vi "Read Buffered Data.vi"(8 "error in (no error)":errorcluster, 11 "Standard Measurement in":refnum<class "Standard Measurement.lvclass">) -> (0 "error out":errorcluster, 3 "Standard Measurement out":refnum<class "Standard Measurement.lvclass">)   [LabVIEW 2026, in "Standard Measurement Plugin.lvlib" / "Standard Measurement.lvclass"]
doc: "Read one snapshot from each configured Standard Measurement hardware buffer and store latest waveforms. Three hardware roles maximum; each preview waits at most 1 ms, zero retries. Incoming errors bypass reads through the framework accessors; timeout or type conversion errors propagate. No hardware initialization or actor launch."
uses:
  Standard Measurement.lvclass
  framework/Measurement Actor/Measurement.lvclass
  framework/Hardware/Hardware.lvclass
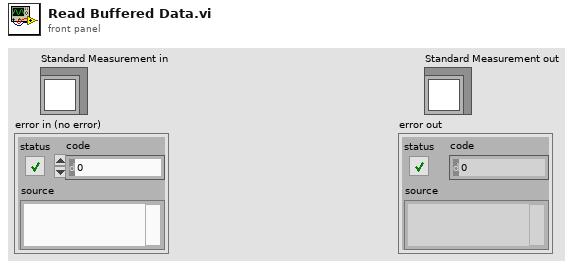
[diagram p1: front panel]
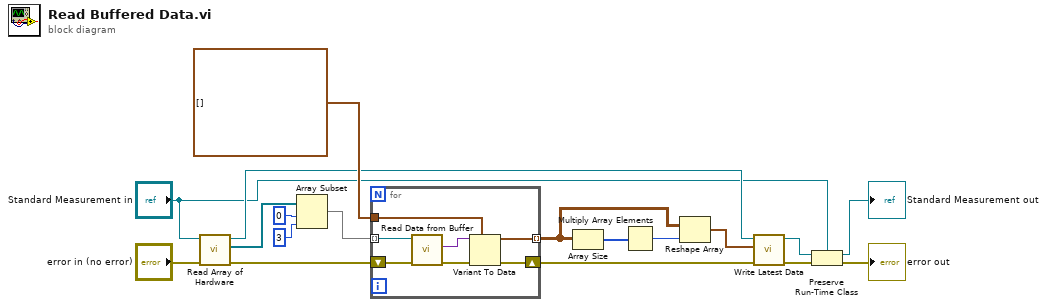
[diagram p0: block diagram]
diagram:
  n1 = call "Read Array of Hardware.vi"("error in (no error)"="error in (no error)", "Measurement in"="Standard Measurement in") -> ("error out"=w12:errorcluster, "Array of Hardware"=w17:refnum<class "Hardware.lvclass">[], "Measurement out"=w8:refnum<class "Standard Measurement.lvclass">)  [unwired: 7 in]
  n2 = Array Subset(array=w17, index=0, length=3) -> (w14:refnum<class "Hardware.lvclass">[])
  n3 = for {
    tunnel: w14 -> [w25] mode=indexing
    tunnel: waveform(dbl)[] [] -> [w22]
    shift-right: [w20] -> w6
    shift-left: w12 -> [w24]
    tunnel: [w19] -> w11 mode=indexing
    n4 = call "Read Data from Buffer.vi"("error in (no error)"=w24, "Hardware in"=w25) -> ("error out"=w21:errorcluster, "Variant"=w23:variant)  [unwired: 7 in, 1 out]
    n5 = Variant To Data(error in=w21, type=w22, Variant=w23) -> (data=w19:waveform(dbl)[], error out=w20:errorcluster)
  }
  n6 = Array Size(array=w11) -> (size(s)=w10:i32[])
  n7 = Multiply Array Elements(1:w10) -> (0:w9:i32)
  n8 = Reshape Array(w11, w9) -> (w7:waveform(dbl)[])
  n9 = call "Write Latest Data.vi"("error in (no error)"=w6, "latest data"=w7, "Measurement in"=w8) -> ("error out"=w3:errorcluster, "Measurement out"=w5:refnum<class "Standard Measurement.lvclass">)  [unwired: 7 in]
  n10 = Preserve Run-Time Class(object in=w5, error in=w3, 2:"Standard Measurement in") -> (object out=→"Standard Measurement out":refnum<class "Standard Measurement.lvclass">, error out=→"error out":errorcluster)
